vi "Close Power Supply.vi"(0 "reference in":refnum<class "Power Supply.lvclass">, 5 "error in (no error)":errorcluster) -> (14 "reference out":refnum<class "Power Supply.lvclass">, 18 "Power Supply Open/Close Status":bool, 19 "error out":errorcluster)   [LabVIEW 2017, in "Power Supply.lvclass"]
uses:
  Power Supply.lvclass
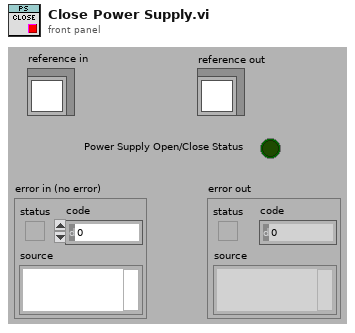
[diagram p1: front panel]
types:
  T1 = typedef "Power Supply.lvclass/ObjectAttributes.ctl" = cluster{"Power Supply Chain VISA Session":refnum<visa-resource-name>, "Power Supply Chain Address":i16, "Power Supply Open/Close Status":bool, "Power Supply Voltage Setting":dbl, "Power Supply Current Setting":dbl, "Power Supply Voltage Reading":dbl, "Power Supply Current Reading":dbl, "Power Supply Status":T2, "Power Supply Error":T3, "Fault Register":u8, "Power Supply Error":bool}
  T2 = typedef "Power Supply.lvclass/Power Supply Status.ctl" = enum16{"Closed", "Open"}
  T3 = typedef "Power Supply.lvclass/Power Supply Error.ctl" = enum16{"None", "Read Error"}
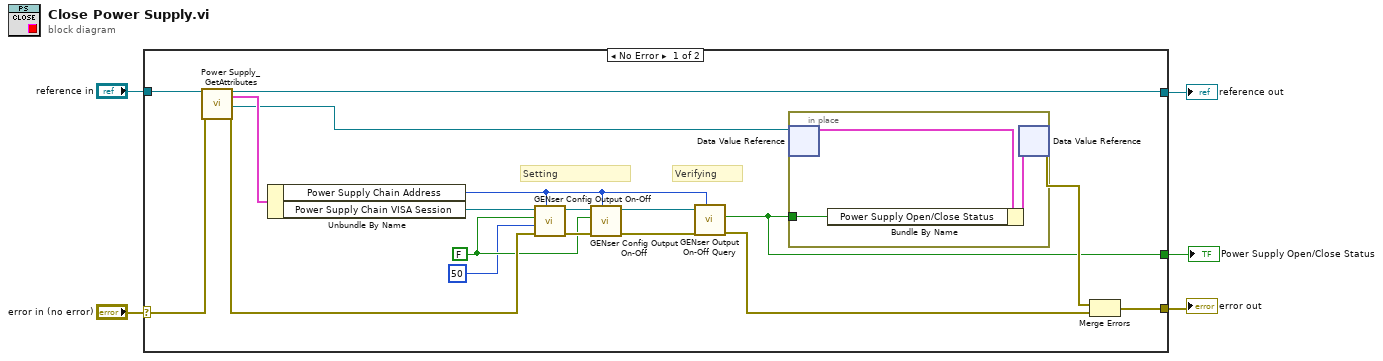
[diagram p0: block diagram]
diagram:
  n1 = case shown="No Error" "error in (no error)" {
    selector: "error in (no error)" -> [w22 w28]
    tunnel: [w18 w28] -> w4
    tunnel: [w19 w27] -> w2
    tunnel: "reference in" -> [w23 w27]
    tunnel: [w6 _] -> w1
    frame No Error {
      w12 = FALSE ("Output ON")
      # "Verifying"
      # "Setting"
      n2 = call "Power Supply_GetAttributes.vi"("reference in"=w23, "error in (no error)"=w22) -> ("reference out"=w19:refnum<class "Power Supply.lvclass">, "Data"=w21:T1, "DataRef"=w17:refnum<data-value>, "error out"=w15:errorcluster)  [unwired: 14 in]
      n3 = Unbundle By Name(w21) -> ("Power Supply Chain Address"=w8:i16, "Power Supply Chain VISA Session"=w16:refnum<visa-resource-name>)
      n4 = call <instrlib>:"GENser Config Output On-Off.vi"("GEN Addr"=w8, "error"=w15, "Settle (0 mS)"=u32 50, "Output ON"=w12, "VISA"=w16) -> ("error out"=w13:errorcluster, "VISA out"=w14:refnum<visa-resource-name>)  [unwired: 5 in]
      n5 = call <instrlib>:"GENser Config Output On-Off.vi"("GEN Addr"=w8, "error"=w13, "Output ON"=w12, "VISA"=w14) -> ("error out"=w9:errorcluster, "VISA out"=w10:refnum<visa-resource-name>)  [unwired: 6 in]
      n6 = call <instrlib>:"GENser Output On-Off Query.vi"("GEN Addr"=w8, "error"=w9, "VISA"=w10) -> ("error out"=w7:errorcluster, "Output ON"=w6:bool)  [unwired: 6 in, 1 out]
      n7 = in-place {
        in-place-border: w6 -> [w24]
        n8 = in-place-dvr #1(w17) -> (w25:T1)  [unwired: 1 out]
        n9 = Bundle By Name(cluster=w25, "Power Supply Open/Close Status"=w24) -> (w26:T1)
        n10 = in-place-dvr #1(w26) -> (w20:errorcluster)  [unwired: 1 out]
      }
      n11 = Merge Errors(w20, w7) -> (w18:errorcluster)
    }
    frame Error {
    }
  }
  "error out" <- w4
  "reference out" <- w2
  "Power Supply Open/Close Status" <- w1
